vi "test_LoadCompiledSettings.vi"() -> ()   [LabVIEW 2020]
uses:
  14a89e45-9281-4f82-9a61-2239173df7bc.vi
  <vilib>/NI VeriStand/Custom Device API/Custom Device Item Ref.ctl
  <vilib>/NI VeriStand/Custom Device API/Custom Device API.lvlib
  Source/Shared/Controls and Global/RT messageType.ctl
  Source/Shared/Ballard 1553 Shared.lvlib
  Source/Shared/Controls and Global/RT CWD1.ctl
  Source/Shared/Controls and Global/RT CWD2.ctl
  <vilib>/NI VeriStand/Custom Device API/Data Reference.ctl
  <vilib>/NI VeriStand/Custom Device API/Block Data Reference.ctl
  Source/Shared/EncodeDecode/_typedefs/parameter_config_type_type.ctl
  Source/Shared/EncodeDecode/_typedefs/parameter_config_encoding_type.ctl
  Source/Shared/EncodeDecode/_typedefs/parameter_config_type.ctl
  Source/Shared/Controls and Global/RT Message.ctl
  Source/Shared/Controls and Global/RT BC.ctl
  Source/Shared/Controls and Global/RT Remote Terminal_rtMode.ctl
  Source/Shared/Controls and Global/RT Remote Terminal_RT direction.ctl
  Source/Shared/Controls and Global/RT Remote Terminal_RT subAddress.ctl
  Source/Shared/Controls and Global/RT Remote Terminal_RT Mode Code.ctl
  Source/Shared/Controls and Global/RT Remote Terminal.ctl
  Source/Shared/Controls and Global/RT Channel.ctl
  Source/Shared/Controls and Global/Compiled.Settings.ctl
panel:
  out "Data out":T1 {"channels"."RTs"."Mode Codes"."Timestamp Channel Data Reference" format="%.0x"; "channels"."RTs"."subAddresses"."Timestamp Channel Data Reference" format="%.0x"; "channels"."RTs"."Status Channel Data Reference" format="%.0x"; "channels"."RTs"."Command Channels Refs" format="%.0x"; "channels"."BC"."Acyclic Frames Trigger Channels Refs" format="%.0x"; "channels"."BC"."Command Channels Refs" format="%.0x"; "channels"."BC"."messages"."Timestamp Channel Data Reference" format="%.0x"; "channels"."BC"."messages"."Status Channel Data Refs" format="%.0x"; "channels"."BC"."messages"."Words Item Refs" format="%.0x"}
  in  "compiled settings json":path
  out "error out":errorcluster
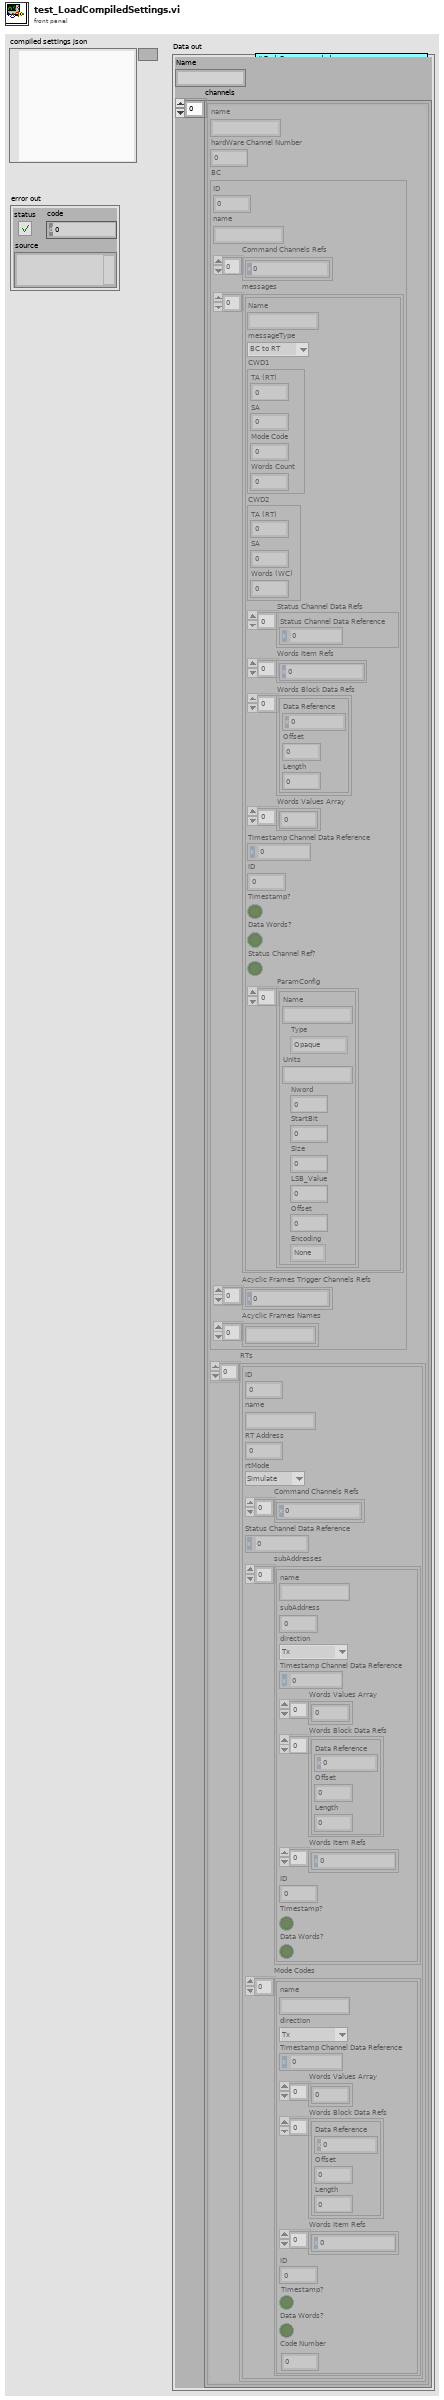
[diagram p1: front panel]
types:
  T1 = typedef "Ballard 1553 Shared.lvlib/Compiled.Settings.ctl" = cluster{"Name":string, "channels":T2[]}
  T2 = typedef "Ballard 1553 Shared.lvlib/RT Channel.ctl" = cluster{"name":string, "hardWare Channel Number":u16, "BC":T3, "RTs":T14[]}
  T3 = typedef "Ballard 1553 Shared.lvlib/RT BC.ctl" = cluster{"ID":i32, "name":string, "Command Channels Refs":T4[], "messages":T5[], "Acyclic Frames Trigger Channels Refs":T4[], "Acyclic Frames Names":string[]}
  T4 = typedef "Custom Device API.lvlib/Custom Device Item Ref.ctl" = u64
  T5 = typedef "Ballard 1553 Shared.lvlib/RT Message.ctl" = cluster{"Name":string, "messageType":T6, "CWD1":T7, "CWD2":T8, "Status Channel Data Refs":T9[], "Words Item Refs":T4[], "Words Block Data Refs":T10[], "Words Values Array":u16[], "Timestamp Channel Data Reference":T9, "ID":i32, "Timestamp?":bool, "Data Words?":bool, "Status Channel Ref?":bool, "ParamConfig":T11[]}
  T6 = typedef "Ballard 1553 Shared.lvlib/RT messageType.ctl" = enum16{"BC to RT", "RT to BC", "RT to RT", "MC (Rx)", "MC (Tx)"}
  T7 = typedef "Ballard 1553 Shared.lvlib/RT CWD1.ctl" = cluster{"TA (RT)":i8, "SA":i8, "Mode Code":i8, "Words Count":i8}
  T8 = typedef "Ballard 1553 Shared.lvlib/RT CWD2.ctl" = cluster{"TA (RT)":i8, "SA":i8, "Words (WC)":i8}
  T9 = typedef "Custom Device API.lvlib/Data Reference.ctl" = i32
  T10 = typedef "Custom Device API.lvlib/Block Data Reference.ctl" = cluster{"Data Reference":T9, "Offset":u64, "Length":u64}
  T11 = typedef "parameter_config_type.ctl" = cluster{"Name":string, "Type":T12, "Units":string, "Nword":i32, "StartBit":i32, "Size":i32, "LSB_Value":i32, "Offset":i32, "Encoding":T13}
  T12 = typedef "parameter_config_type_type.ctl" = enum16{"Opaque", "Enum", "Float", "Integer", "Bcd", "Bool"}
  T13 = typedef "parameter_config_encoding_type.ctl" = enum16{"None", "2-complement", "Unsigned"}
  T14 = typedef "Ballard 1553 Shared.lvlib/RT Remote Terminal.ctl" = cluster{"ID":i32, "name":string, "RT Address":i32, "rtMode":T15, "Command Channels Refs":T4[], "Status Channel Data Reference":T9, "subAddresses":T16[], "Mode Codes":T18[]}
  T15 = typedef "Ballard 1553 Shared.lvlib/RT Remote Terminal_rtMode.ctl" = enum16{"Simulate", "Monitor", "Disable"}
  T16 = typedef "Ballard 1553 Shared.lvlib/RT Remote Terminal_RT subAddress.ctl" = cluster{"name":string, "subAddress":i8, "direction":T17, "Timestamp Channel Data Reference":T9, "Words Values Array":u16[], "Words Block Data Refs":T10[], "Words Item Refs":T4[], "ID":i32, "Timestamp?":bool, "Data Words?":bool}
  T17 = typedef "Ballard 1553 Shared.lvlib/RT Remote Terminal_RT direction.ctl" = enum16{"Tx", "Rx"}
  T18 = typedef "Ballard 1553 Shared.lvlib/RT Remote Terminal_RT Mode Code.ctl" = cluster{"name":string, "direction":T17, "Timestamp Channel Data Reference":T9, "Words Values Array":u16[], "Words Block Data Refs":T10[], "Words Item Refs":T4[], "ID":i32, "Timestamp?":bool, "Data Words?":bool, "Code Number":i32}
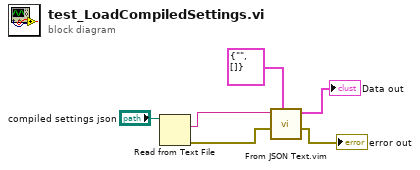
[diagram p0: block diagram]
diagram:
  n1 = Read from Text File(file (use dialog)="compiled settings json") -> (text=w6:string, error out=w5:errorcluster)  [unwired: 3 in, 2 out]
  n2 = call "From JSON Text.vim"("Data Type and Default Value"=T1 {"Name"="", "channels"=[]} ("Compiled.Settings"), "error in (no error)"=w5, "JSON"=w6) -> ("error out"=→"error out":errorcluster, "Data out"=→"Data out":T1)  [unwired: 7 in]
